vi "Write Log.vi"(10 "Log entry":string, 11 "SolutionBuilder in":refnum<class "SolutionBuilder.lvclass">) -> (3 "SolutionBuilder out":refnum<class "SolutionBuilder.lvclass">)   [LabVIEW 2020, in "SolutionBuilder.lvlib" / "SolutionBuilder.lvclass"]
uses:
  SolutionBuilder.lvclass
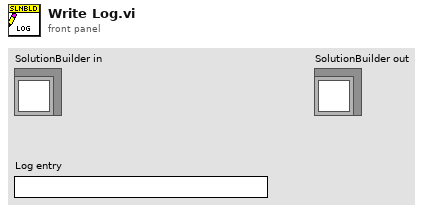
[diagram p1: front panel]
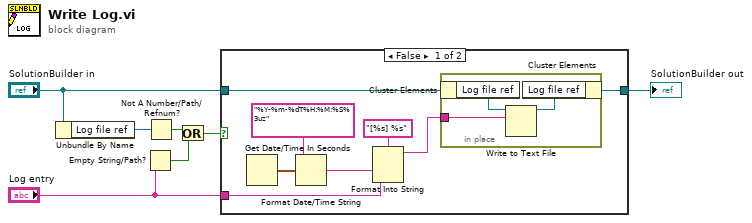
[diagram p0: block diagram]
diagram:
  n1 = Unbundle By Name("SolutionBuilder in") -> ("Log file ref"=w4:refnum<file>)
  n2 = Empty String/Path?(string/path="Log entry") -> (empty?=w2:bool)
  n3 = Not A Number/Path/Refnum?(number/path/refnum=w4) -> (NaN/Path/Refnum?=w3:bool)
  n4 = Or(x=w3, y=w2) -> (x .or. y?=w1:bool)
  n5 = case shown="False" w1 {
    tunnel: "SolutionBuilder in" -> [w15 w19]
    tunnel: "Log entry" -> [w9 _]
    tunnel: [w14 w19] -> w6
    frame False {
      n6 = Get Date/Time In Seconds() -> (seconds since 1Jan1904=w12:timestamp)
      n7 = Format Date/Time String(time format string (%c)="%Y-%m-%dT%H:%M:%S%3uz", seconds (now)=w12) -> (date/time string=w11:string)  [unwired: 1 in]
      n8 = Format Into String(format string="[%s] %s", w11, w9) -> (resulting string=w8:string)  [unwired: 2 in, 1 out]
      n9 = in-place {
        in-place-border: w8 -> [w16]
        n10 = in-place-cluster #1(w15) -> ("Log file ref"=w18:refnum<file>)
        n11 = Write to Text File(file (use dialog)=w18, text=w16) -> (refnum out=w17:refnum<file>)  [unwired: 2 in, 2 out]
        n12 = in-place-cluster #1("Log file ref"=w17) -> (w14:refnum<class "SolutionBuilder.lvclass">)
      }
    }
    frame True {
    }
  }
  "SolutionBuilder out" <- w6
